vi "ConfigureChannelProperties.vi"(5 "fpga tach buffer multiplier":i32, 6 "Channels per Dynamic Module":i32[](array[numeric])=[3, 3, 3, 4, 4], 7 "fpga tach buffer minimum":i32, 8 "error in (no error)":errorcluster, 9 "Sampling Rate":dbl format="%#_13g", 10 "Filtered Channels (in acquisition order)":T10[](array[typedef])) -> (0 "error out":errorcluster, 2 "valid":bool, 3 "acq config":T1 {"HighPassFilterState"."Filter State" format="%.2f"; "HighPassFilterState"."IIR Filter Cluster"."Forward Coefficients" format="%.2f"; "HighPassFilterState"."IIR Filter Cluster"."Reverse Coefficients" format="%.2f"; "FixedSizeX32"."InputConfig" items=["AC Coupled", "DC Coupled", "IEPE AC Coupled"]})   [LabVIEW 2017, in "CmsAcquisition.lvlib"]
uses:
  <vilib>/addons/InsightCM/Devices/Shared/Cms/CmsAcquisition/CmsAcquisition.lvlib
  <vilib>/addons/InsightCM/MessageBus/Base/controls/R2_Channel.ctl
  <vilib>/addons/InsightCM/MessageBus/Base/controls/KeyValuePair.ctl
  <vilib>/addons/InsightCM/MessageBus/Base/controls/Metric.ctl
  <vilib>/addons/InsightCM/Devices/Shared/Cms/CmsAcquisition/controls/Configuration.ctl
  <vilib>/addons/InsightCM/Devices/Shared/Cms/CmsAcquisition/controls/TachometerConfig.ctl
  <vilib>/addons/InsightCM/Devices/Shared/Cms/CmsAcquisition/controls/FixedSizeArrays.ctl
  <vilib>/LabVIEW Targets/FPGA/cRIO/shared/nicrio_ModuleControls/nicrio_cRIO-9232_ConfigModeRing.ctl
  <vilib>/addons/InsightCM/Devices/Shared/Cms/cRIOWfmAcq/subVIs/RIO Wfm Cust Ctrls/rwfm_SamplingInfo.ctl
  <vilib>/addons/InsightCM/Devices/Shared/Cms/CmsAcquisition/controls/Group.ctl
  <vilib>/addons/InsightCM/Devices/Shared/Cms/CmsAcquisition/controls/Channel.ctl
  <vilib>/addons/InsightCM/Utilities/Analysis/Vibration/controls/HighPassFilterState.ctl
  <vilib>/addons/InsightCM/Devices/Shared/Cms/CmsAcquisition/controls/BurstMode.ctl
  <vilib>/addons/InsightCM/Devices/Shared/Cms/cRIOWfmAcq/cRIOWfmLib.lvlib
  <vilib>/addons/InsightCM/Utilities/PropertyHelpers/PropertyHelpers.lvlib
  <vilib>/addons/InsightCM/Utilities/Analysis/Vibration/VibrationAnalysisFunctions.lvlib
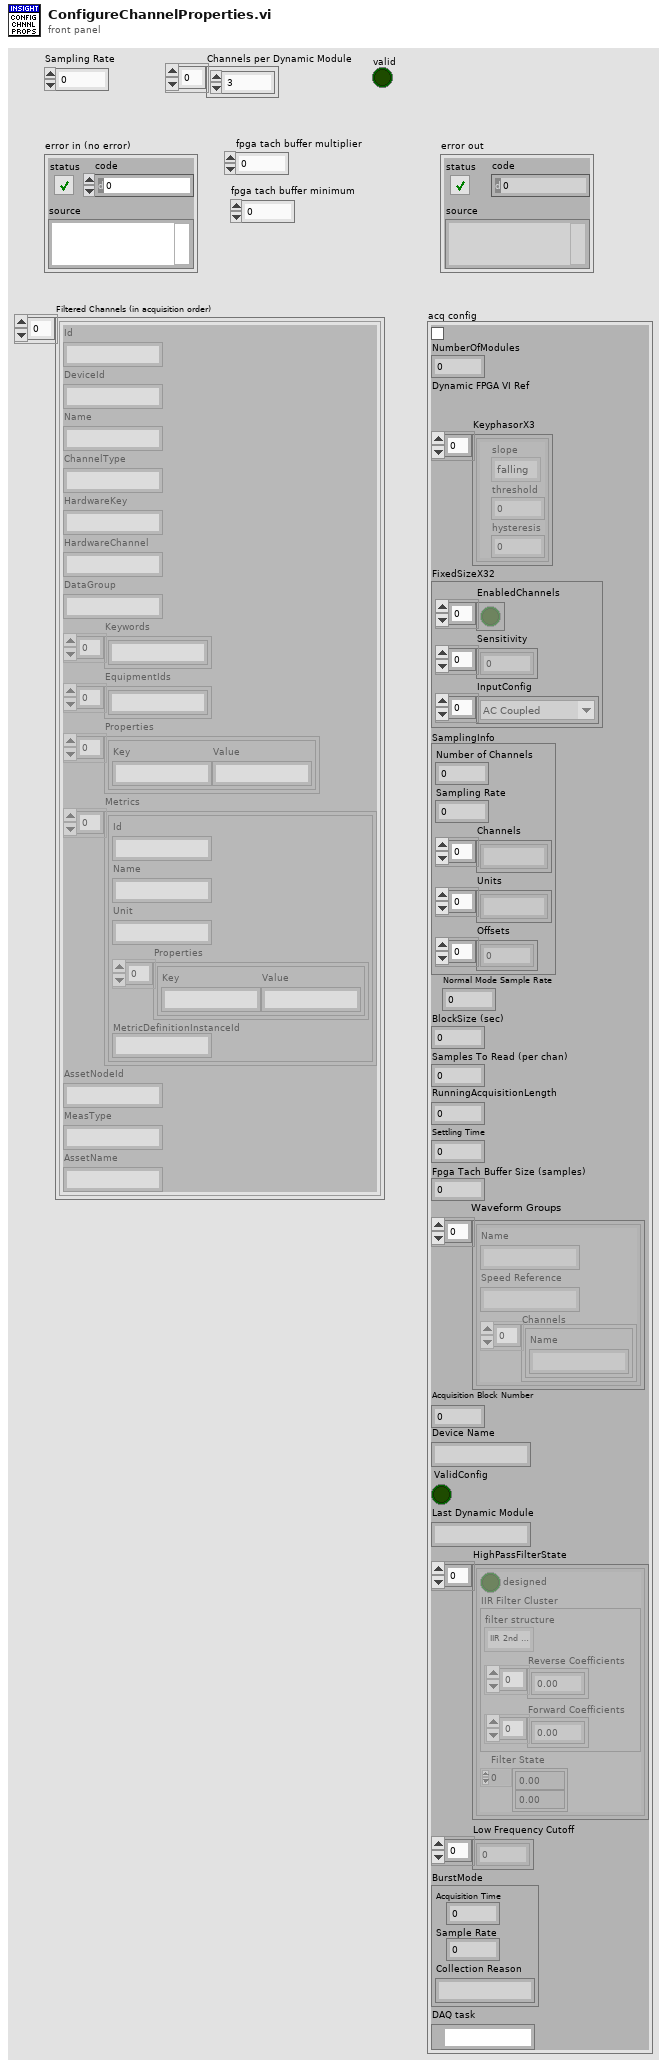
[diagram p1: front panel]
types:
  T1 = typedef "CmsAcquisition.lvlib/Configuration.ctl" = cluster{"Acq":bool, "NumberOfModules":i16, "Dynamic FPGA VI Ref":refnum<k20>, "KeyphasorX3":T2[], "FixedSizeX32":T3, "SamplingInfo":T5, "Normal Mode Sample Rate":dbl, "BlockSize (sec)":dbl, "Samples To Read (per chan)":i32, "RunningAcquisitionLength":dbl, "Settling Time":dbl, "Fpga Tach Buffer Size (samples)":i32, "Waveform Groups":T6[], "Acquisition Block Number":i32, "Device Name":string, "ValidConfig":bool, "Last Dynamic Module":string, "HighPassFilterState":T8[], "Low Frequency Cutoff":dbl[], "BurstMode":T9, "DAQ task":refnum<k21>}
  T2 = typedef "CmsAcquisition.lvlib/TachometerConfig.ctl" = cluster{"slope":enum16{"falling", "rising"}, "threshold":dbl, "hysteresis":dbl}
  T3 = typedef "CmsAcquisition.lvlib/FixedSizeArrays.ctl" = cluster{"EnabledChannels":bool[], "Sensitivity":dbl[], "InputConfig":T4[]}
  T4 = typedef "nicrio_cRIO-9232_ConfigModeRing.ctl" = u8
  T5 = typedef "cRIOWfmLib.lvlib/rwfm_SamplingInfo.ctl" = cluster{"Number of Channels":i32, "Sampling Rate":dbl, "Channels":string[], "Units":string[], "Offsets":sgl[]}
  T6 = typedef "CmsAcquisition.lvlib/Group.ctl" = cluster{"Name":string, "Speed Reference":string, "Channels":T7[]}
  T7 = typedef "CmsAcquisition.lvlib/Channel.ctl" = cluster{"Name":string}
  T8 = typedef "VibrationAnalysisFunctions.lvlib/HighPassFilterState.ctl" = cluster{"designed":bool, "IIR Filter Cluster":cluster{"filter structure":enum32{"IIR 2nd Order", "IIR 4th Order"}, "Reverse Coefficients":dbl[], "Forward Coefficients":dbl[]}, "Filter State":dbl[]}
  T9 = typedef "CmsAcquisition.lvlib/BurstMode.ctl" = cluster{"Acquisition Time":dbl, "Sample Rate":dbl, "Collection Reason":string}
  T10 = typedef "R2_Channel.ctl" = cluster{"Id":string, "DeviceId":string, "Name":string, "ChannelType":string, "HardwareKey":string, "HardwareChannel":string, "DataGroup":string, "Keywords":string[], "EquipmentIds":string[], "Properties":T11[], "Metrics":T12[], "AssetNodeId":string, "MeasType":string, "AssetName":string}
  T11 = typedef "KeyValuePair.ctl" = cluster{"Key":string, "Value":string}
  T12 = typedef "Metric.ctl" = cluster{"Id":string, "Name":string, "Unit":string, "Properties":T11[], "MetricDefinitionInstanceId":string}
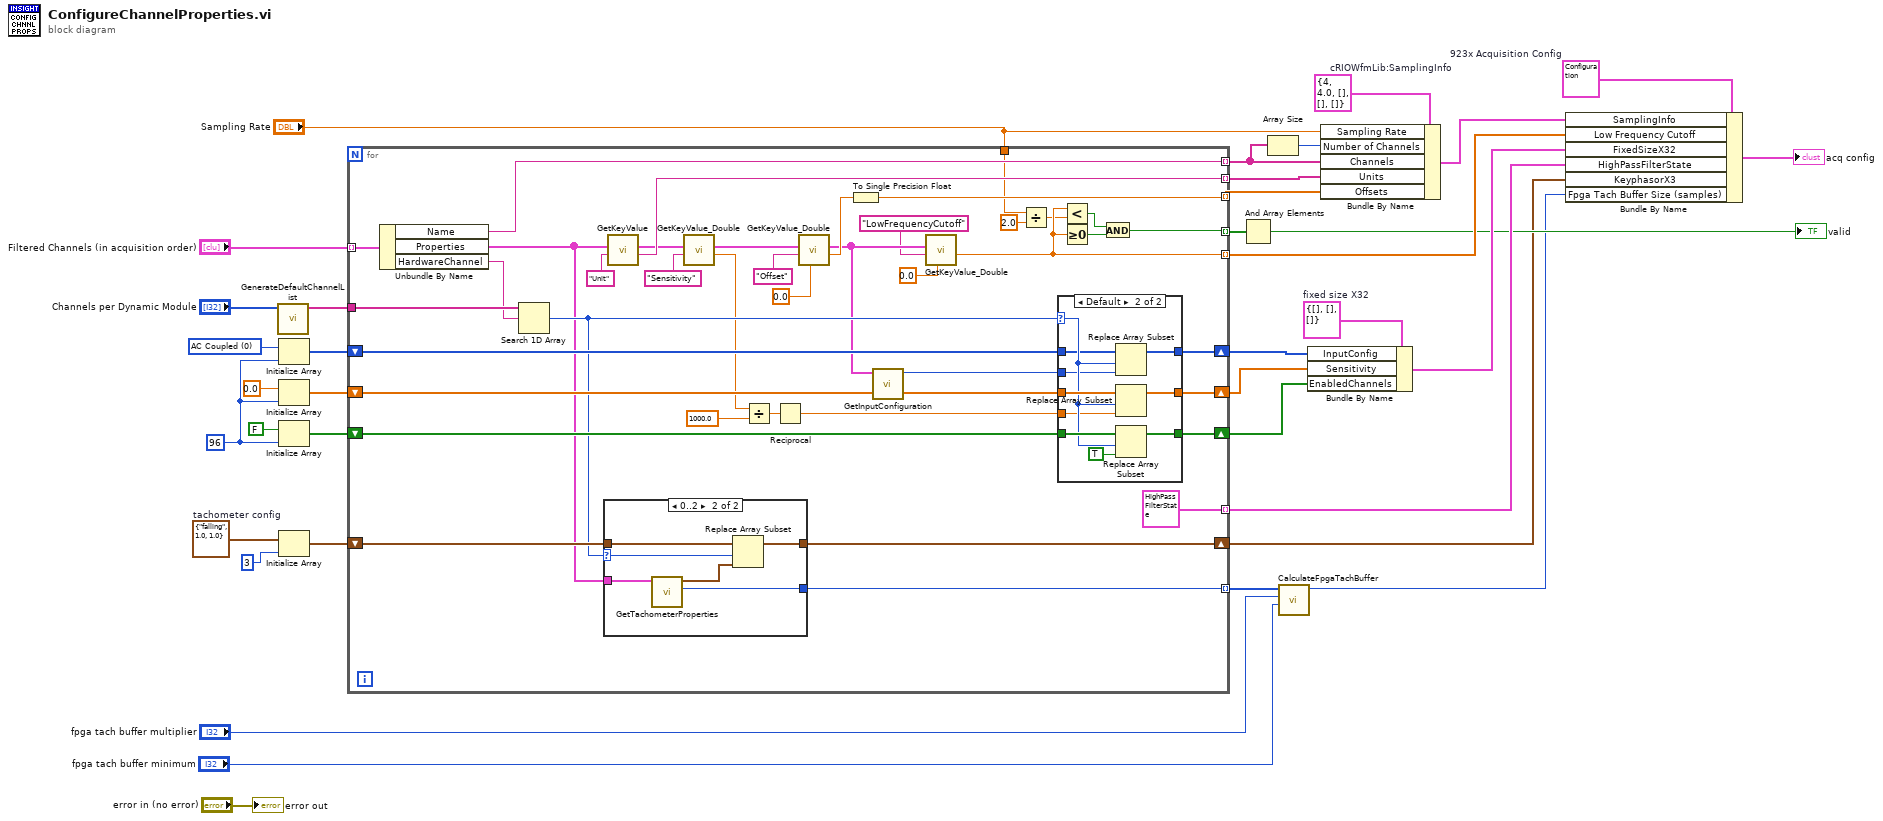
[diagram p0: block diagram]
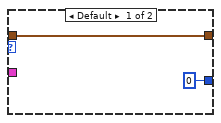
[diagram p2: hidden frame]
diagram:
  w14 = T1 {"Acq"=FALSE, "NumberOfModules"=0, "Dynamic FPGA VI Ref"=refnum, "KeyphasorX3"=[], "FixedSizeX32"={"EnabledChannels"=[], "Sensitivity"=[], "InputConfig"=[]}, "SamplingInfo"={"Number of Channels"=4, "Sampling Rate"=4.0, "Channels"=[], "Units"=[], "Offsets"=[]}, "Normal Mode Sample Rate"=0.0, "BlockSize (sec)"=0.0, "Samples To Read (per chan)"=0, "RunningAcquisitionLength"=0.0, "Settling Time"=0.0, "Fpga Tach Buffer Size (samples)"=0, "Waveform Groups"=[], "Acquisition Block Number"=0, "Device Name"="", "ValidConfig"=FALSE, "Last Dynamic Module"="", "HighPassFilterState"=[], "Low Frequency Cutoff"=[], "BurstMode"={"Acquisition Time"=0.0, "Sample Rate"=0.0, "Collection Reason"=""}, "DAQ task"=""}  # 923x Acquisition Config
  w21 = T5 {"Number of Channels"=4, "Sampling Rate"=4.0, "Channels"=[], "Units"=[], "Offsets"=[]}  # cRIOWfmLib:SamplingInfo
  w37 = T2 {"slope"=enum."falling", "threshold"=1.0, "hysteresis"=1.0}  # tachometer config
  w32 = T3 {"EnabledChannels"=[], "Sensitivity"=[], "InputConfig"=[]}  # fixed size X32
  w28 = T4 0 items=["AC Coupled", "DC Coupled", "IEPE AC Coupled"] ("Input_Configuration")
  w29 = 96 ("dimension size")
  n1 = call <vilib>:"GenerateDefaultChannelList.vi"("Channels per Dynamic Module"="Channels per Dynamic Module") -> ("default channel list"=w22:string[])  [unwired: 10 in]
  n2 = Initialize Array(w28, w29) -> (w31:T4[])
  n3 = Initialize Array(0.0 ("value"), w29) -> (w30:dbl[])
  n4 = Initialize Array(FALSE, w29) -> (w26:bool[])
  n5 = Initialize Array(w37, 3 ("dimension size")) -> (w24:T2[])
  n6 = for {
    tunnel: "Filtered Channels (in acquisition order)" -> [w69] mode=indexing
    shift-right: [w76] -> w35
    shift-left: w26 -> [w77]
    shift-right: [w74] -> w5
    shift-left: w24 -> [w75]
    shift-right: [w72] -> w34
    shift-left: w30 -> [w73]
    shift-right: [w70] -> w33
    shift-left: w31 -> [w71]
    tunnel: w22 -> [w68]
    tunnel: [w66] -> w19 mode=indexing
    tunnel: [w58] -> w20 mode=indexing
    tunnel: [w50] -> w15 mode=indexing
    tunnel: [T8 {"designed"=FALSE, "IIR Filter Cluster"={"filter structure"=enum."IIR 2nd Order", "Reverse Coefficients"=[], "Forward Coefficients"=[]}, "Filter State"=[]} ("Highpass Filter State")] -> w10 mode=indexing
    tunnel: [w43] -> w12 mode=indexing
    tunnel: "Sampling Rate" -> [w41]
    tunnel: [w39] -> w7 mode=indexing
    tunnel: [w38] -> w4 mode=indexing
    n7 = Unbundle By Name(w69) -> ("Name"=w66:string, "Properties"=w60:T11[], "HardwareChannel"=w67:string)
    n8 = Search 1D Array(1D array=w68, element=w67) -> (index of element=w65:i32)  [unwired: 1 in]
    n9 = case shown="0..2" w65 {
      selector: w65 -> [_ w84]
      tunnel: w75 -> [w79 w85]
      tunnel: [w79 w83] -> w74
      tunnel: w60 -> [_ w82]
      tunnel: [0 ("pulses per rev") w80] -> w38
      frame Default {
      }
      frame 0..2 {
        n10 = call <vilib>:"GetTachometerProperties.vi"("Properties"=w82) -> ("pulses per rev"=w80:i32, "Tachometer Config"=w81:T2)  [unwired: 8 in, 1 out]
        n11 = Replace Array Subset(array=w85, new element=w81, index=w84) -> (w83:T2[])
      }
    }
    n12 = call <vilib>:"GetKeyValue.vi"("key"="Unit" ("name"), "key value pairs"=w60) -> ("value"=w58:string, "key value pairs out"=w57:T11[])  [unwired: 7 in, 1 out]
    n13 = call <vilib>:"GetKeyValue_Double.vi"("key"="Sensitivity" ("name"), "key value pairs"=w57) -> ("value"=w55:dbl, "key value pairs out"=w53:T11[])  [unwired: 7 in, 1 out]
    n14 = Divide(x=w55, y=1000.0) -> (x/y=w62:dbl)
    n15 = Reciprocal(x=w62) -> (1/x=w61:dbl)
    n16 = call <vilib>:"GetKeyValue_Double.vi"("default"=0.0, "key"="Offset" ("name"), "key value pairs"=w53) -> ("value"=w51:dbl, "key value pairs out"=w48:T11[])  [unwired: 6 in, 1 out]
    n17 = To Single Precision Float(number=w51) -> (single precision float=w50:sgl)
    n18 = call <vilib>:"GetInputConfiguration.vi"("Properties"=w48) -> ("Input Configuration"=w64:T4)  [unwired: 10 in]
    n19 = call <vilib>:"GetKeyValue_Double.vi"("default"=0.0, "key"="LowFrequencyCutoff", "key value pairs"=w48) -> ("value"=w43:dbl)  [unwired: 6 in, 2 out]
    n20 = Divide(x=w41, y=2.0) -> (x/y=w42:dbl)
    n21 = case shown="Default" w65 {
      selector: w65 -> [_ w94]
      tunnel: w77 -> [w88 w98]
      tunnel: [w88 w96] -> w76
      tunnel: w73 -> [w86 w95]
      tunnel: [w86 w93] -> w72
      tunnel: w71 -> [w87 w92]
      tunnel: [w87 w91] -> w70
      tunnel: w64 -> [_ w90]
      tunnel: w61 -> [_ w89]
      frame -1 {
      }
      frame Default {
        n22 = Replace Array Subset(array=w92, new element=w90, index=w94) -> (w91:T4[])
        n23 = Replace Array Subset(array=w95, new element=w89, index=w94) -> (w93:dbl[])
        n24 = Replace Array Subset(array=w98, new element=TRUE, index=w94) -> (w96:bool[])
      }
    }
    n25 = Less?(x=w43, y=w42) -> (x < y?=w44:bool)
    n26 = Greater Or Equal To 0?(x=w43) -> (x >= 0?=w45:bool)
    n27 = And(x=w44, y=w45) -> (x .and. y?=w39:bool)
  }
  n28 = And Array Elements(Boolean array=w7) -> (logical AND=→"valid":bool)
  n29 = Array Size(array=w19) -> (size(s)=w18:i32)
  n30 = call <vilib>:"CalculateFpgaTachBuffer.vi"("fpga tach buffer minimum"="fpga tach buffer minimum", "fpga tach buffer multiplier"="fpga tach buffer multiplier", "pulses per rev"=w4) -> ("Fpga Tach Buffer Size (samples)"=w3:i32)  [unwired: 8 in]
  n31 = Bundle By Name(cluster=w32, "InputConfig"=w33, "Sensitivity"=w34, "EnabledChannels"=w35) -> (w11:T3)
  n32 = Bundle By Name(cluster=w21, "Sampling Rate"="Sampling Rate", "Number of Channels"=w18, "Channels"=w19, "Units"=w20, "Offsets"=w15) -> (w13:T5)
  n33 = Bundle By Name(cluster=w14, "SamplingInfo"=w13, "Low Frequency Cutoff"=w12, "FixedSizeX32"=w11, "HighPassFilterState"=w10, "KeyphasorX3"=w5, "Fpga Tach Buffer Size (samples)"=w3) -> (→"acq config":T1)
  "error out" <- "error in (no error)"
